vi "OneStep.vi"(8 "error in (no error)":errorcluster, 11 "StepperMotor in":refnum<class "StepperMotor.lvclass">) -> (0 "error out":errorcluster, 3 "StepperMotor out":refnum<class "StepperMotor.lvclass">)   [LabVIEW 2022 SP3, in "Motorshield.lvlib" / "StepperMotor.lvclass"]
uses:
  StepperMotor.lvclass
  StepperMotor.lvclass/StepperMotor.ctl
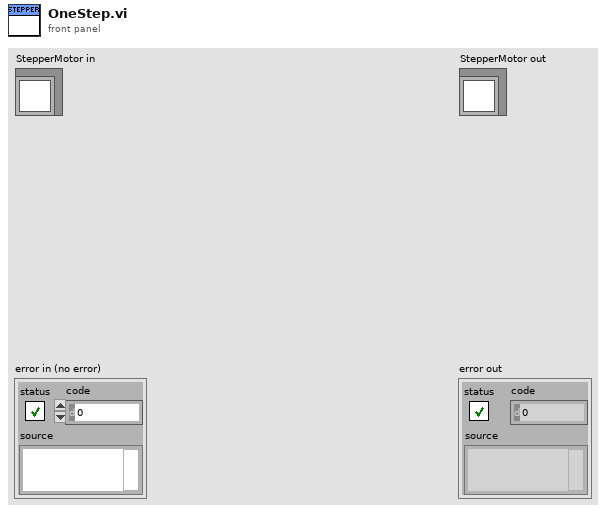
[diagram p1: front panel]
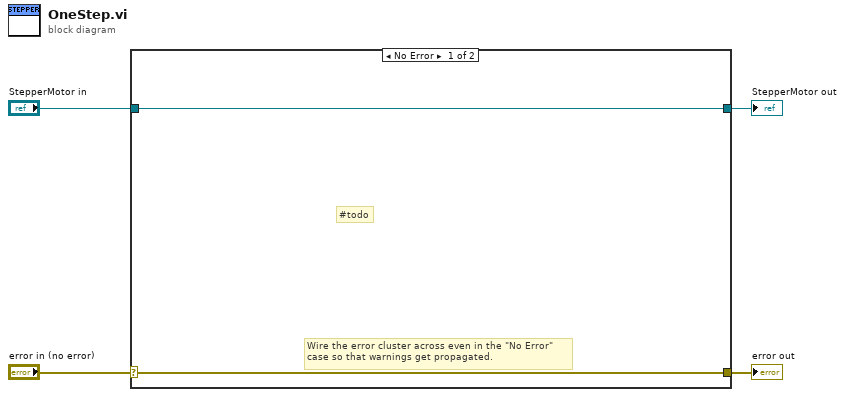
[diagram p0: block diagram]
diagram:
  n1 = case shown="No Error" "error in (no error)" {
    selector: "error in (no error)" -> [w5 w8]
    tunnel: [w5 w8] -> w3
    tunnel: [w6 w7] -> w1
    tunnel: "StepperMotor in" -> [w6 w7]
    frame No Error {
      # "#todo"
      # "Wire the error cluster across even in the \"No Error\"\ncase so that warnings get propagated."
    }
    frame Error {
    }
  }
  "error out" <- w3
  "StepperMotor out" <- w1
